vi "LVClass_ModalCoef GetZernikePrefs.vi"(0 "ModalCoef in":refnum<class "ModalCoef.lvclass">, 11 "error in (no error)":errorcluster) -> (4 "ModalCoef out":refnum<class "ModalCoef.lvclass">, 6 "ZernikeModalPrefs":T1={"Number of coefficients"=32, "Filtered coefficients"=[], "RMS Zernike normalization"=FALSE, "CircularProjectionPupilDimensions"={"Pupil center_sspp"={"X"=0.0, "Y"=0.0}, "Pupil radius_sspp"=0.0}}, 10 "nb_polynomial_base_to_filter":u32, 15 "error out":errorcluster)   [LabVIEW 2020, in "ModalCoef.lvclass"]
doc: "Get preferences for phase reconstruction from Zernike decomposition.\n\n--------------------------------------------------------------------------------\n\n<B>ComputePhaseSetIn </B> : ComputePhaseSet object.\n<B>ComputePhaseSetOut </B> : ComputePhaseSet object.\n<B>normalisation </B> : Normalisation Phase coefficients enumeration :\n * 0 : standard\n * 1 : rms\n<B>nb_coeffs_total </B> : Number of the Zernike coefficients used in the polynomial base.\n<B>nb_coeffs_to_filter </B> : Number of the Zernike coefficients to filter in the polynomial base.\n<B>coeffs_to_filter </B> : Indices of the Zernike coefficients to filter in the polynomial base.\n<B>projection_pupil_center </B> : Center of the projection pupil, in number of subpupils.\n<B>projection_pupil_radius </B> : Projection pupil radius, in number of subpupils.\n<B>ErrorIn </B> : Error\n<B>ErrorOut </B> : Error\n\n--------------------------------------------------------------------------------"
uses:
  ModalCoef.lvclass
  Controls/ZernikeModalPrefs.ctl
  Controls/ZernikeProjectionPupilSetup.ctl
  Controls/Point2Df.ctl
  ModalCoef.lvclass/ModalCoef.ctl
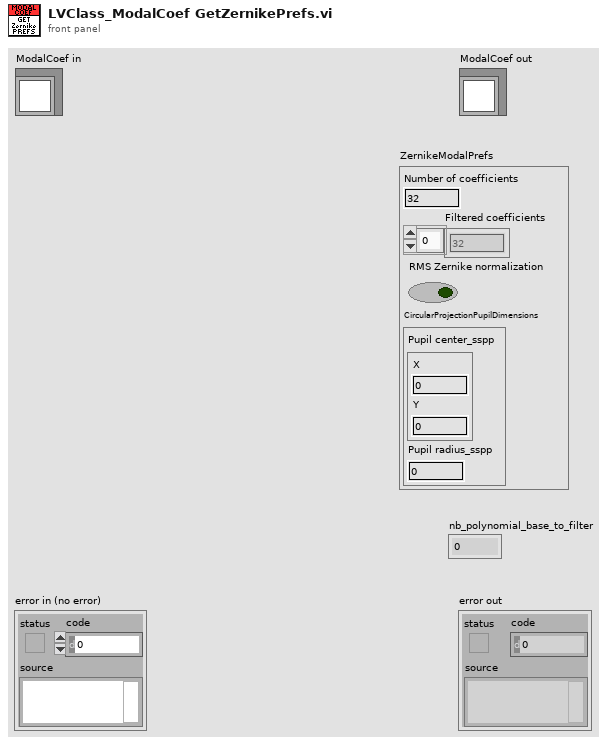
[diagram p1: front panel]
types:
  T1 = typedef "ZernikeModalPrefs.ctl" = cluster{"Number of coefficients":u32, "Filtered coefficients":u32[], "RMS Zernike normalization":bool, "CircularProjectionPupilDimensions":T2}
  T2 = typedef "ZernikeProjectionPupilSetup.ctl" = cluster{"Pupil center_sspp":T3, "Pupil radius_sspp":sgl}
  T3 = typedef "Point2Df.ctl" = cluster{"X":sgl, "Y":sgl}
  T4 = typedef "ClassID.ctl" = i64
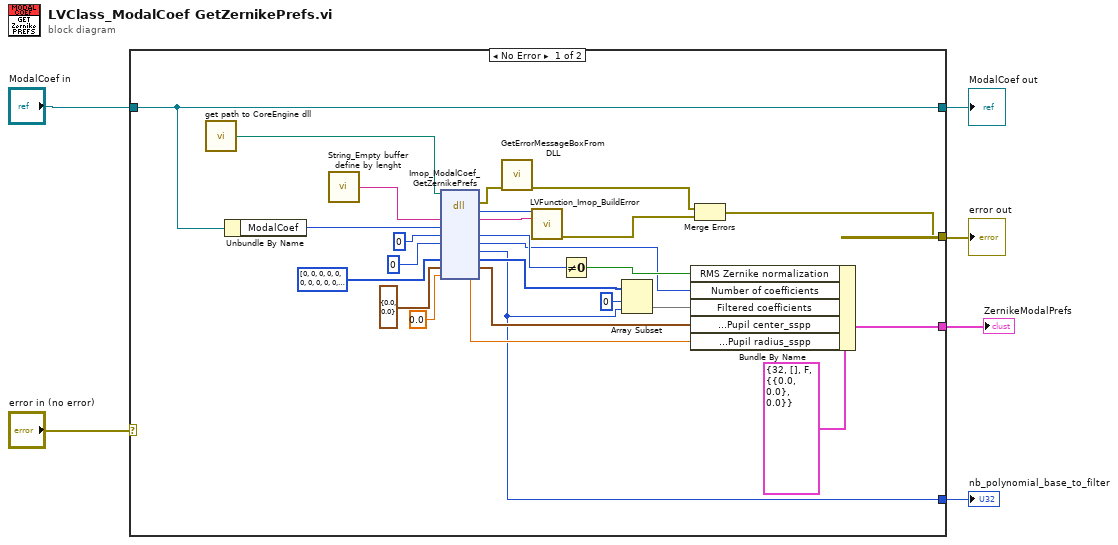
[diagram p0: block diagram]
diagram:
  n1 = case shown="No Error" "error in (no error)" {
    selector: "error in (no error)" -> [_ w34]
    tunnel: [w7 w34] -> w3
    tunnel: [w12 w33] -> w5
    tunnel: "ModalCoef in" -> [w12 w33]
    tunnel: [w26 _] -> w2
    tunnel: [w10 _] -> w1
    frame No Error {
      n2 = call "get path to CoreEngine dll.vi"() -> ("path to wavekit library"=w29:path)  [unwired: 14 in, 1 out]
      n3 = Unbundle By Name(w12) -> ("ModalCoef"=w11:T4)
      n4 = call "String_Empty buffer define by lenght.vi"() -> ("Empty buffer"=w30:string)  [unwired: 1 in]
      n5 = dll-call lib="D:/2_trunk/Soft_haso/ImOpCoreEngine4_LV2011/DLLs/ImopEngine4_vc100.dll" fn="Imop_ModalCoef_GetZernikePrefs"(path in=w29, "message"=w30, "objet"=w11, "normalisation"=u8 0, "numberOfCoefficient"=u32 0, "polynomial_base"=u32[] [0, 0, 0, 0, 0, 0, 0, 0, 0, 0, 0, 0, 0, 0, 0, 0, 0, 0, 0, 0, 0, 0, 0, 0, 0, 0, 0, 0, 0, 0, 0, 0, 0, 0, 0, 0, 0, 0, 0, 0, 0, 0, 0, 0, 0, 0, 0, 0, 0, 0, 0, 0, 0, 0, 0, 0, 0, 0, 0, 0, 0, 0, 0, 0, 0, 0, 0, 0, 0, 0, 0, 0, 0, 0, 0, 0, 0, 0, 0, 0, 0, 0, 0, 0, 0, 0, 0, 0, 0, 0, 0, 0, 0, 0, 0, 0, 0, 0, 0, 0, 0, 0, 0, 0, 0, 0, 0, 0, 0, 0, 0, 0, 0, 0, 0, 0, 0, 0, 0, 0, 0, 0, 0, 0, 0, 0, 0, 0, 0], "projection_pupil_center"=T3 {"X"=0.0, "Y"=0.0} ("CircularProjectionPupilDimensions.Pupil center_sspp"), "projection_pupil_diameter"=sgl 0.0) -> (error out=w28:errorcluster, "return type"=w32:i32, "message"=w31:string, "normalisation"=w20:u8, "numberOfCoefficient"=w15:u32, "nb_polynomial_base_to_filter"=w10:u32, "polynomial_base"=w14:u32[], "projection_pupil_center"=w18:T3, "projection_pupil_diameter"=w17:sgl)  [unwired: 4 in, 1 out]
      n6 = call "GetErrorMessageBoxFromDLL.vi"("error IN"=w28) -> ("error OUT"=w9:errorcluster)  [unwired: 10 in]
      n7 = call "LVFunction_Imop_BuildError.vi"("code"=w32, "String to Prepend to source (\"\")"=w31) -> ("error out"=w8:errorcluster)  [unwired: 13 in]
      n8 = Not Equal To 0?(x=w20) -> (x != 0?=w19:bool)
      n9 = Array Subset(array=w14, index=0, length=w10) -> (w13:u32[])
      n10 = Bundle By Name(cluster=T1 {"Number of coefficients"=32, "Filtered coefficients"=[], "RMS Zernike normalization"=FALSE, "CircularProjectionPupilDimensions"={"Pupil center_sspp"={"X"=0.0, "Y"=0.0}, "Pupil radius_sspp"=0.0}} ("ZernikeModalPrefs"), "RMS Zernike normalization"=w19, "Number of coefficients"=w15, "Filtered coefficients"=w13, "CircularProjectionPupilDimensions.Pupil center_sspp"=w18, "CircularProjectionPupilDimensions.Pupil radius_sspp"=w17) -> (w26:T1)
      n11 = Merge Errors(w9, w8) -> (w7:errorcluster)
    }
    frame Error {
    }
  }
  "error out" <- w3
  "ModalCoef out" <- w5
  "ZernikeModalPrefs" <- w2
  "nb_polynomial_base_to_filter" <- w1
